vi "Caller_Method.vi"(0 "Object In":refnum<class "Arithmetic_Operations.lvclass">, 11 "Error In":errorcluster) -> (4 "Object Out":refnum<class "Arithmetic_Operations.lvclass">, 15 "Error Out":errorcluster)   [LabVIEW 2020]
uses:
  Arithmetic_Operations.lvclass
  Children/Add/Add.lvclass
  D:/Github Projects/LV_Assignment/Tasks/A17/Calculator_using_instance/Classes/Arithmetic_Operations/Arithmetic_Operations.lvclass
  Children/Add/Methods/UI.vi
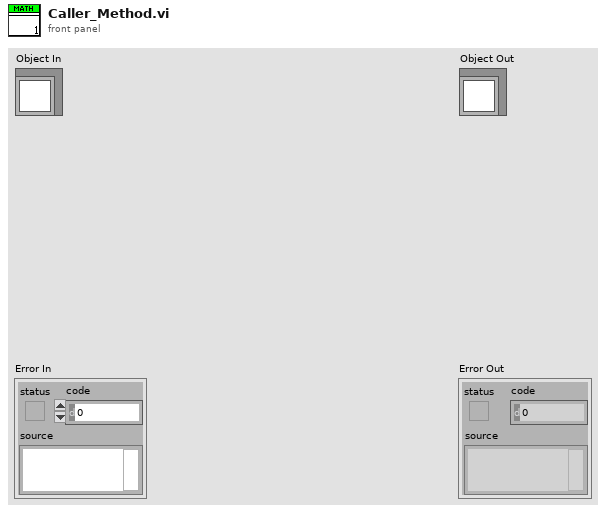
[diagram p1: front panel]
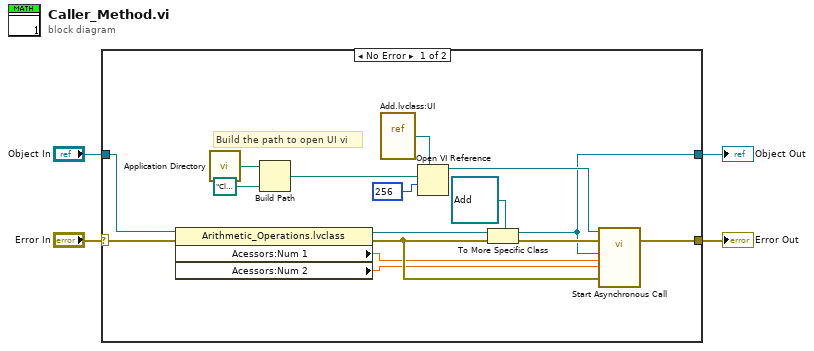
[diagram p0: block diagram]
diagram:
  n1 = case shown="No Error" "Error In" {
    selector: "Error In" -> [w7 w22]
    tunnel: [w8 w22] -> w3
    tunnel: [w5 w21] -> w1
    tunnel: "Object In" -> [w6 w21]
    frame No Error {
      # "Build the path to open UI vi"
      n2 = property class="Arithmetic_Operations.lvclass"(reference=w6, error in=w7) -> (reference out=w9:refnum<class "Arithmetic_Operations.lvclass">, error out=w20:errorcluster, "Acessors:Num 1"=w13:dbl, "Acessors:Num 2"=w12:dbl)
      n3 = call <vilib>:"Application Directory.vi"() -> ("Application Directory"=w15:path)
      n4 = Build Path(base path=w15, name or relative path=path "Classes/Children/Add/Methods/UI.vi") -> (appended path=w16:path)
      n5 = vi-ref "Add.lvclass:UI.vi"() -> (w19:refnum<vi>)
      n6 = Open VI Reference(type specifier VI Refnum (for type only)=w19, vi path=w16, options=256) -> (vi reference=w17:refnum<vi>)  [unwired: 3 in, 1 out]
      n7 = To More Specific Class(target class=refnum<class "Add.lvclass"> refnum ("Add.lvclass"), reference=w9, error in=w20) -> (specific class reference=w5:refnum<class "Add.lvclass">, error out=w11:errorcluster)
      n8 = call-by-ref "Start Asynchronous Call"(reference=w17, error in=w11, "Add.lvclass"=w5, "Num 1"=w13, "Num 2"=w12, "Error In"=w20) -> (error out=w8:errorcluster)  [unwired: 9 in, 4 out]
    }
    frame Error {
    }
  }
  "Error Out" <- w3
  "Object Out" <- w1
